vi "Update Command Status.vi"(8 "error in (no error)":errorcluster, 10 "Command Status":T1, 11 "Command Actor in":refnum<class "Command Actor.lvclass">) -> (0 "error out":errorcluster, 3 "Command Actor out":refnum<class "Command Actor.lvclass">)   [LabVIEW 2013, in "Command Actor.lvlib" / "Command Actor.lvclass"]
uses:
  Command Actor.lvclass
  Command/Command Status.ctl
  Command/Command States.ctl
  Command/State Status.ctl
  Command Actor.lvclass/Command Actor.ctl
  Command/Command State Actor.lvclass
  Command States/Command States.lvclass
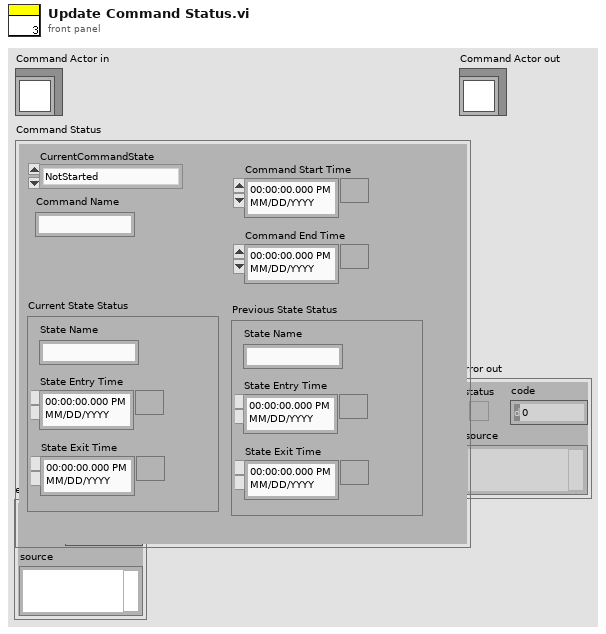
[diagram p1: front panel]
types:
  T1 = typedef "Command State Actor.lvlib/Command State Actor.lvclass/Command Status.ctl" = cluster{"CurrentCommandState":T2, "Command Name":string, "Current State Status":T3, "Command Start Time":timestamp, "Command End Time":timestamp, "Previous State Status":T3}
  T2 = typedef "Command State Actor.lvlib/Command State Actor.lvclass/Command States.ctl" = enum16{"NotStarted", "Starting", "Started", "Executing", "Completing", "Completed", "Stopping", "Stopped"}
  T3 = typedef "Command Actor.lvlib/Command States.lvclass/State Status.ctl" = cluster{"State Name":string, "State Entry Time":timestamp, "State Exit Time":timestamp}
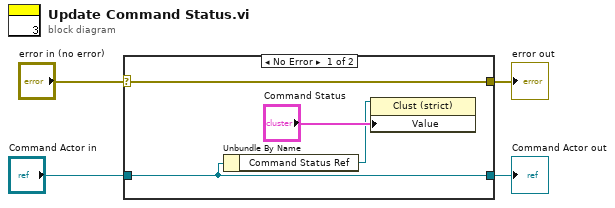
[diagram p0: block diagram]
diagram:
  n1 = case shown="No Error" "error in (no error)" {
    selector: "error in (no error)" -> [w8 w10]
    tunnel: [w8 w10] -> w3
    tunnel: [w7 w9] -> w1
    tunnel: "Command Actor in" -> [w7 w9]
    frame No Error {
      n2 = Unbundle By Name(w7) -> ("Command Status Ref"=w5:refnum<vi>)
      n3 = property class="Clust (strict)"(reference=w5, "Value"="Command Status") -> ()  [unwired: 1 in, 2 out]
    }
    frame Error {
    }
  }
  "error out" <- w3
  "Command Actor out" <- w1
